vi "Drivebase Tele-Op.vi"(9 "Buttons":bool[](array[boolean]), 10 "Axes":dbl[](array[numeric])) -> ()   [LabVIEW 2019]
uses:
  3cacb506-33a2-4e6e-84d7-2b7690206a7b.vi
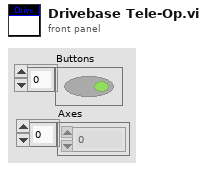
[diagram p1: front panel]
types:
  T1 = cluster{"Left Motor Value":dbl, "Right Motor Value":dbl}
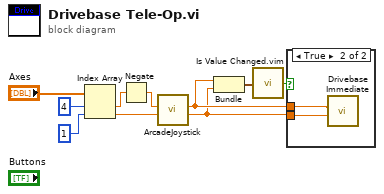
[diagram p0: block diagram]
diagram:
  n1 = Index Array(array="Axes", index #1=4 ("index"), index #2=1 ("index")) -> (element #1=w2:dbl, element #2=w7:dbl)
  n2 = Negate(x=w2) -> (-x=w1:dbl)
  n3 = call "ArcadeJoystick.vi"("Y axis value"=w7, "X axis value"=w1) -> ("Right Motor Value"=w4:dbl, "Left Motor Value"=w5:dbl)  [unwired: 8 in]
  n4 = Bundle("Left Motor Value"=w5, "Right Motor Value"=w4) -> (w6:T1)  [unwired: 1 in]
  n5 = call "Is Value Changed.vim"("value"=w6) -> ("changed or first call?"=w3:bool)
  n6 = case shown="True" w3 {
    tunnel: w5 -> [_ w12]
    tunnel: w4 -> [_ w11]
    frame False {
    }
    frame True {
      n7 = call "Drivebase Immediate.vi"("Left Setpoint"=w11, "Right Setpoint"=w12) -> ()  [unwired: 10 in]
    }
  }
